vi "ClosestPoint.vi"(6 "Reset":bool, 8 "Robot":cluster{"x":dbl, "y":dbl}, 11 "Path":cluster{"x":dbl, "y":dbl}[](array[cluster])) -> (2 "ClosestIndex":i32, 3 "Point":cluster{"x":dbl, "y":dbl})   [LabVIEW 2020]
doc: "Find the closest point to the robot"
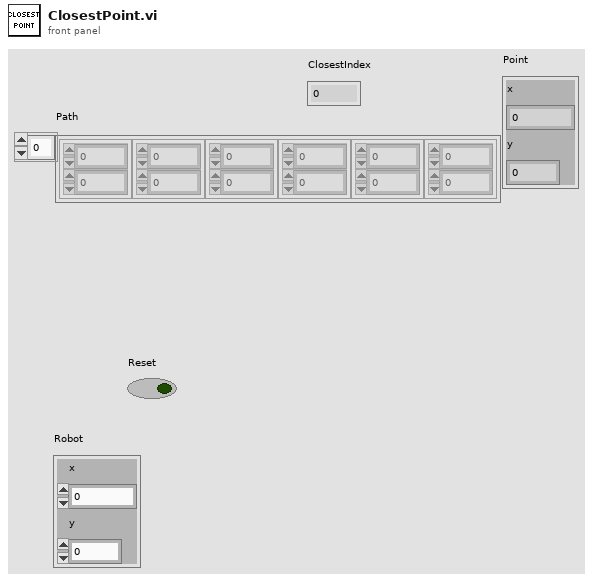
[diagram p1: front panel]
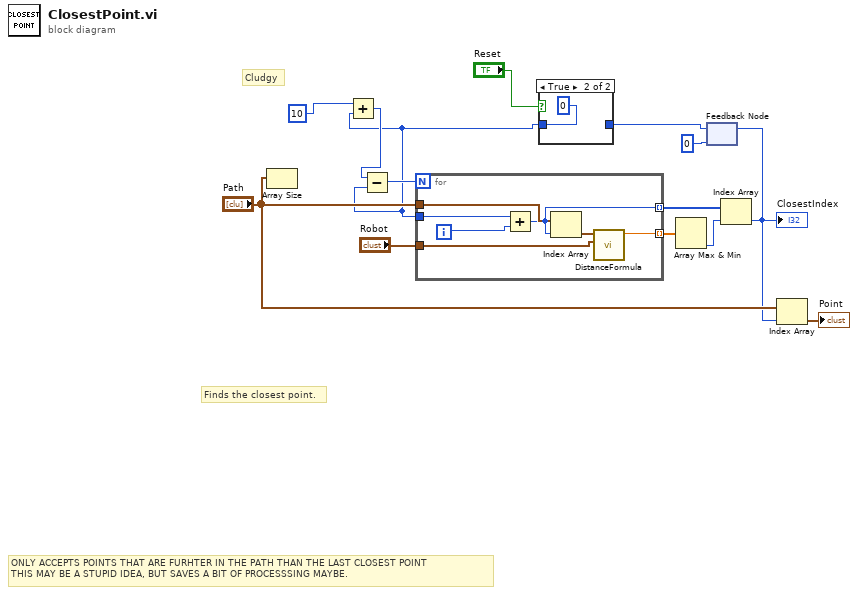
[diagram p0: block diagram]
diagram:
  # "Cludgy"
  # "ONLY ACCEPTS POINTS THAT ARE FURHTER IN THE PATH THAN THE LAST CLOSEST POINT\nTHIS MAY BE A STUPID IDEA, BUT SAVES A BIT OF PROCESSSING MAYBE."
  # "Finds the closest point."
  n1 = Array Size(array="Path") -> ()  [unwired: 1 out]
  n2 = feedback #1(0) -> (w2:i32)
  n3 = case shown="True" "Reset" {
    tunnel: w2 -> [w15 _]
    tunnel: [w15 0] -> w1
    frame False {
    }
    frame True {
    }
  }
  n4 = Add(x=10, y=w1) -> (x+y=w5:i32)
  n5 = Subtract(x=w5, y=w1) -> (x-y=w10:i32)
  n6 = for {
    N: w10 -> [_]
    tunnel: "Path" -> [w22]
    tunnel: "Robot" -> [w23]
    tunnel: w1 -> [w21]
    tunnel: [w19] -> w8 mode=indexing
    tunnel: [w18] -> w9 mode=indexing
    i -> [w17]
    n7 = Add(x=w21, y=w17) -> (x+y=w19:i32)
    n8 = Index Array(array=w22, index=w19) -> (element=w20:cluster{"x":dbl, "y":dbl})
    n9 = call "DistanceFormula.vi"("Point 2"=w23, "Point 1"=w20) -> ("Distance"=w18:dbl)  [unwired: 9 in]
  }
  n10 = Array Max & Min(array=w9) -> (min index (indices)=w7:i32)  [unwired: 3 out]
  n11 = Index Array(array=w8, index=w7) -> (element=w3:i32)
  "ClosestIndex" <- w3
  n12 = feedback-in #1(w3) -> ()
  n13 = Index Array(array="Path", index=w3) -> (element=→"Point":cluster{"x":dbl, "y":dbl})
